vi "L01.vi"() -> ()   [LabVIEW 2012]
panel:
  out "sum":i32
  out "Array":i32[](array[numeric])
  in  "Numeric":i32
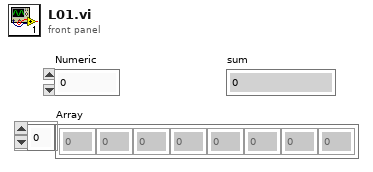
[diagram p1: front panel]
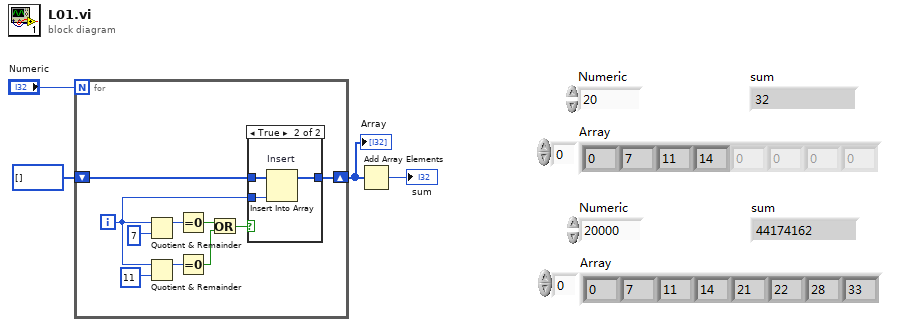
[diagram p0: block diagram]
diagram:
  n1 = for {
    N: "Numeric" -> [_]
    shift-right: [w7] -> w2
    shift-left: i32[] [] -> [w6]
    i -> [w5]
    n2 = Quotient & Remainder(x=w5, y=7) -> (x-y*floor(x/y)=w11:i32)  [unwired: 1 out]
    n3 = Quotient & Remainder(x=w5, y=11) -> (x-y*floor(x/y)=w12:i32)  [unwired: 1 out]
    n4 = Equal To 0?(x=w11) -> (x = 0?=w9:bool)
    n5 = Equal To 0?(x=w12) -> (x = 0?=w10:bool)
    n6 = Or(x=w9, y=w10) -> (x .or. y?=w8:bool)
    n7 = case shown="True" w8 {
      tunnel: [w15 w18] -> w7
      tunnel: w6 -> [w15 w17]
      tunnel: w5 -> [_ w16]
      frame False {
      }
      frame True {
        n8 = Insert Into Array "Insert"(array=w17, new element=w16) -> (w18:i32[])  [unwired: 1 in]
      }
    }
  }
  "Array" <- w2
  n9 = Add Array Elements(numeric array=w2) -> (sum=→"sum":i32)
